vi "PXI-2514 RT Driver VI.vi"(6 "Device Clock":string, 9 "Device Inputs FIFO":refnum<k33>, 10 "Device Outputs FIFO":refnum<k33>, 11 "Device Reference":T1 format="%.0x") -> ()   [LabVIEW 2011, in "PXI-2514 Custom Device.lvlib"]
uses:
  PXI-2514 Custom Device.lvlib
  <vilib>/NI Veristand/Custom Device API/Custom Device Item Ref.ctl
  <vilib>/NI Veristand/Custom Device API/Custom Device Channel Type.ctl
  <vilib>/Platform/TimedLoop/XDataNode/timing_clust.ctl
  <vilib>/Platform/TimedLoop/XDataNode/nitl_modes.ctl
  <vilib>/Platform/TimedLoop/XDataNode/wakeup.ctl
  FIU Global Strings.vi
  <vilib>/NI Veristand/Custom Device API/Get Item Property (String).vi
  <vilib>/Platform/TimedLoop/XDataNode/XDataNode.xnode
  <vilib>/Platform/TimedLoop/XDataNode/XDNodeRunTimeDep.lvlib
  <vilib>/NI Veristand/Custom Device API/Custom Device API.lvlib
panel:
  in  "Status Notifier":refnum<notifier>
  # "Custom Device Template\nv1.0"
  # "Use this template as a starting point for creating a custom device code module. The input controls shown here are specially named controls that the system will use to provide the device loop with data. The controls are not required for the device loop to run. For instance, if the device doesn't produce any output data, then you don't need the Device Outputs FIFO control. If you do use these controls, however, they need to have these exact names to be functional."
  # "The optional status notifier element is used to notify the RT engine of the last state of the custom device, and to indicate the device has completed execution. If this control is not used, a default No Error value is returned to the system when the device finishes execution."
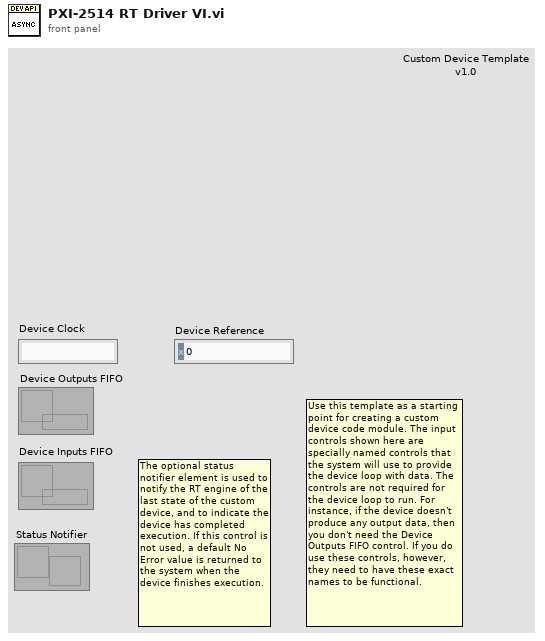
[diagram p1: front panel]
types:
  T1 = typedef "Custom Device API.lvlib/Custom Device Item Ref.ctl" = u64
  T2 = typedef "Custom Device API.lvlib/Custom Device Channel Type.ctl" = enum16{"Input", "Output"}
  T3 = typedef "Custom Device API.lvlib/Custom Device Timed Loop Priority.ctl" = enum32{"Low", "Medium", "High"}
  T4 = typedef "XDNodeRunTimeDep.lvlib/timing_clust.ctl" = cluster{"Expected End [f-1]":u64, "Actual End [f-1]":u64, "Finished Late? [f-1]":bool, "Expected End [i-1]":u64, "Actual End [i-1]":u64, "Finished Late? [i-1]":bool, "Expected Start [i]":u64, "Actual Start [i]":u64, "Expected Start [f]":u64, "Actual Start [f]":u64, "Source Name":string, "Structure Name":string, "Period":i64, "Deadline":i64, "Offset":i64, "Start":i64, "Priority":i32, "Timeout":i32, "Mode":T5, "Wakeup Reason":T6, "Error":errorcluster, "Source Type":string, "Secondary Source Type":string, "Global End Time":u64, "Global Start Time":u64, "Frame Duration":u64, "Iteration Duration":u64, "Assigned CPU":i32, "I/O Scan Engine Mode":u32}
  T5 = typedef "XDNodeRunTimeDep.lvlib/nitl_modes.ctl" = enum32{"No Change", "Process missed periods, maintain original phase", "Discard missed periods, maintain original phase", "Process missed periods, ignore original phase", "Discard missed periods, ignore original phase"}
  T6 = typedef "XDNodeRunTimeDep.lvlib/wakeup.ctl" = enum32{"Normal", "Aborted", "Asynchronous wakeup", "Timing source error", "Timed loop error", "Timeout"}
  T7 = enum16{"Default", "DUT Pass Through", "DUT Open", "DUT Pass Through and FB A", "DUT Pass Through and FB B", "DUT FB A", "DUT FB B"}
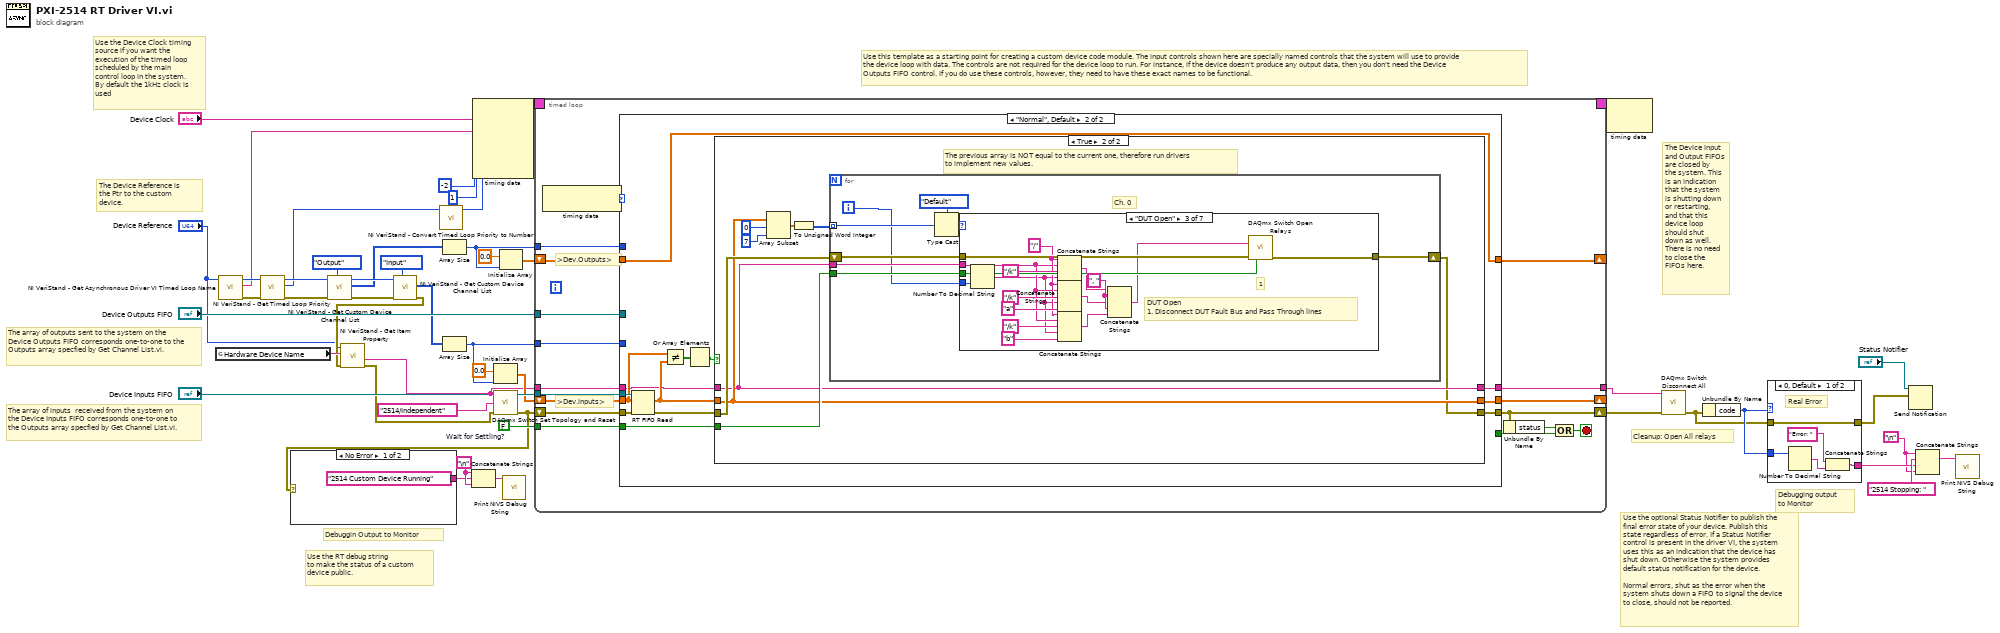
[diagram p0: block diagram]
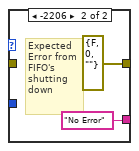
[diagram p2: hidden frame]
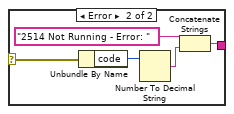
[diagram p3: hidden frame]
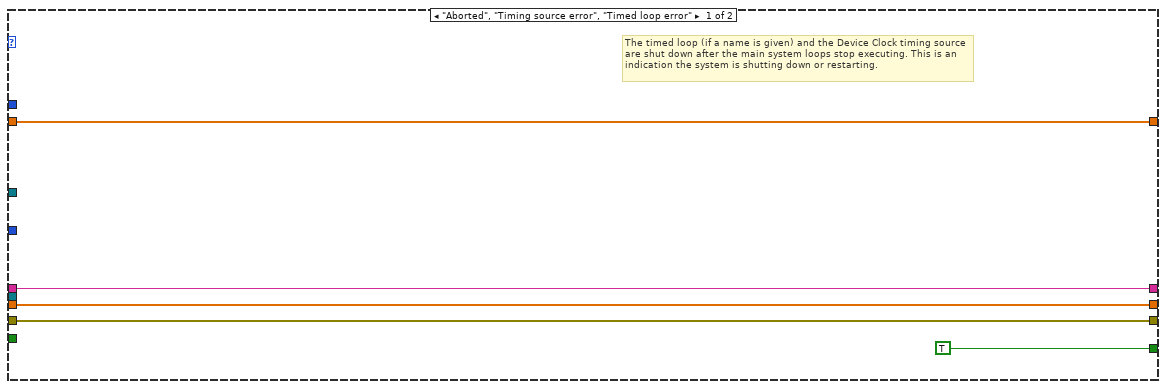
[diagram p4: hidden frame]
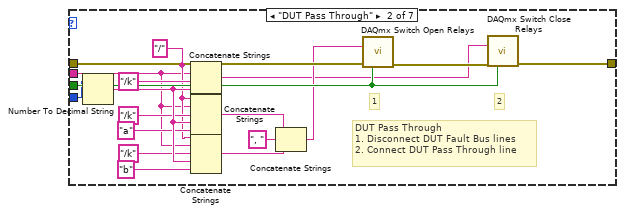
[diagram p7: hidden frame]
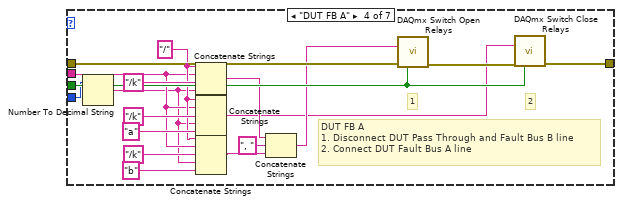
[diagram p8: hidden frame]
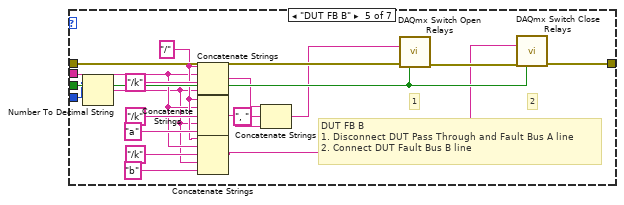
[diagram p9: hidden frame]
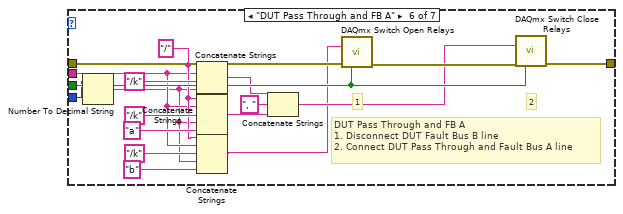
[diagram p10: hidden frame]
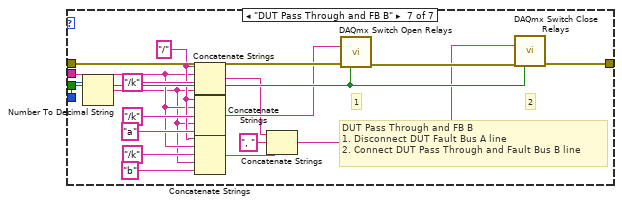
[diagram p11: hidden frame]
diagram:
  w6 = "\n"
  w19 = "\n"
  w22 = FALSE  # Wait for Settling?
  # "Debugging output\nto Monitor"
  # "Debuggin Output to Monitor"
  # "Use the RT debug string\nto make the status of a custom\ndevice public."
  # "Cleanup: Open All relays"
  # "The array of inputs  received from the system on the Device Inputs FIFO corresponds one-to-one to the Outputs array specfied by Get Channel List.vi."
  # "Use the optional Status Notifier to publish the final error state of your device. Publish this state regardless of error. If a Status Notifier control is present in the driver VI, the system uses this as an indication that the device has shut down. Otherwise the system provides default status notification for the device.\n\nNormal errors, shut as the error when the system shuts down a FIFO to signal the device to close, should not be reported."
  # "The Device Input and Output FIFOs are closed by the system. This is an indication that the system is shutting down or restarting, and that this device loop should shut down as well. There is no need to close the FIFOs here."
  # "The array of outputs sent to the system on the Device Outputs FIFO corresponds one-to-one to the Outputs array specfied by Get Channel List.vi."
  # "The Device Reference is\nthe Ptr to the custom device."
  # "Use the Device Clock timing source if you want the execution of the timed loop scheduled by the main control loop in the system. \nBy default the 1kHz clock is used"
  # "Use this template as a starting point for creating a custom device code module. The input controls shown here are specially named controls that the system will use to provide the device loop with data. The controls are not required for the device loop to run. For instance, if the device doesn't produce any output data, then you don't need the Device Outputs FIFO control. If you do use these controls, however, they need to have these exact names to be functional."
  n1 = global read "FIU Global Strings.vi" "Hardware Device Name"() -> (w16:string)
  n2 = call <vilib>:"NI VeriStand - Get Asynchronous Driver VI Timed Loop Name.vi"("Device Ref in"="Device Reference") -> ("error out"=w30:errorcluster, "Device Timed Loop Name"=w36:string, "Device Ref out"=w47:T1)  [unwired: 1 in, 7 out]
  n3 = call <vilib>:"NI VeriStand - Get Timed Loop Priority.vi"("error in (no error)"=w30, "Device Ref in"=w47) -> ("error out"=w31:errorcluster, "Priority"=w27:T3, "Device Ref out"=w32:T1)  [unwired: 7 out]
  n4 = call <vilib>:"NI VeriStand - Get Custom Device Channel List.vi"("Channel Type"=Custom_Device_Channel_Type."Output", "error in (no error)"=w31, "Device Ref in"=w32) -> ("error out"=w35:errorcluster, "Specified Channel Ref List"=w28:T1[], "Device Ref out"=w37:T1)  [unwired: 6 out]
  n5 = call <vilib>:"NI VeriStand - Get Custom Device Channel List.vi"("Channel Type"=Custom_Device_Channel_Type."Input", "error in (no error)"=w35, "Device Ref in"=w37) -> ("error out"=w15:errorcluster, "Specified Channel Ref List"=w29:T1[])  [unwired: 7 out]
  n6 = call-poly <vilib>:"NI VeriStand - Get Item Property.vi"("error in (no error)"=w15, "Property Name"=w16, "Item Ref in"="Device Reference") -> ("error out"=w14:errorcluster, "Value"=w13:string)  [unwired: 5 in, 2 out]
  n7 = call <vilib>:"NI VeriStand - Convert Timed Loop Priority to Number.vi"("Priority"=w27) -> ("Numeric Priority"=w26:i32)  [unwired: 10 out]
  n8 = Array Size(array=w28) -> (size(s)=w33:i32)
  n9 = Array Size(array=w29) -> (size(s)=w23:i32)
  n10 = node-c288("Device Clock", w36, -2 ("Processor"), i64 1 ("Period"), w26) -> (w44:T4)
  n11 = Initialize Array(0.0 ("element"), w23) -> (w39:dbl[])
  n12 = call <vilib>:"DAQmx Switch Set Topology and Reset.vi"("switch device"=w13, "topology name"="2514/Independent" ("string"), "error in"=w14) -> ("error out"=w12:errorcluster)  [unwired: 12 out]
  n13 = case shown="No Error" w12 {
    selector: w12 -> [_ w49]
    tunnel: ["2514 Custom Device Running" ("String to write") w50] -> w18
    frame No Error {
    }
    frame Error {
      n14 = Unbundle By Name(w49) -> ("code"=w53:i32)
      n15 = Number To Decimal String(number=w53) -> (decimal integer string=w51:string)  [unwired: 1 in]
      n16 = Concatenate Strings("2514 Not Running - Error: " ("String to write"), w51) -> (w50:string)
    }
  }
  n17 = Concatenate Strings(w19, w18, w19) -> (w17:string)
  n18 = Initialize Array(0.0 ("element"), w33) -> (w40:dbl[])
  n19 = call "Print NIVS Debug String.vi"("Debug String"=w17) -> ()  [unwired: 9 in, 1 out]
  n20 = timed-loop {
    timing: w44 -> [_]
    timing-out: [_] -> w43
    shift-right: [w68] -> _
    shift-left: w39 -> [w69]
    shift-right: [w61] -> w21
    shift-left: w12 -> [w70]
    shift-right: [w65] -> _
    shift-left: w40 -> [w66]
    tunnel: w33 -> [w62]
    tunnel: "Device Outputs FIFO" -> [w64]
    tunnel: "Device Inputs FIFO" -> [w63]
    tunnel: w23 -> [w57]
    tunnel: w22 -> [w56]
    tunnel: w13 -> [w55]
    tunnel: [w54] -> w20
    stop <- w58 stop-if-true
    # ">Dev.Outputs>"
    # ">Dev.Inputs>"
    n21 = node-c288() -> (w67:T6)  [unwired: 1 out]
    n22 = case shown="\"Normal\", Default" w67 {
      tunnel: w70 -> [w74 w82]
      tunnel: w69 -> [w75 w80]
      tunnel: [w74 w88] -> w61
      tunnel: [w75 w79] -> w68
      tunnel: w66 -> [w73 w78]
      tunnel: [w73 w78] -> w65
      tunnel: w64 -> [_ _]
      tunnel: w63 -> [_ w81]
      tunnel: w62 -> [_ _]
      tunnel: [TRUE _] -> w59
      tunnel: w57 -> [_ _]
      tunnel: w56 -> [_ w87]
      tunnel: w55 -> [w71 w77]
      tunnel: [w71 w76] -> w54
      frame "Aborted", "Timing source error", "Timed loop error" {
        # "The timed loop (if a name is given) and the Device Clock timing source are shut down after the main system loops stop executing. This is an indication the system is shutting down or restarting."
      }
      frame "Normal", Default {
        n23 = RT FIFO Read(0:w81, 1:w80, 3:w82) -> (9:w83:dbl[], 11:w85:errorcluster)  [unwired: 4 out]
        n24 = Not Equal?(x=w80, y=w83) -> (x != y?=w86:bool[])
        n25 = Or Array Elements(Boolean array=w86) -> (logical OR=w84:bool)
        n26 = case shown="True" w84 {
          tunnel: [w90 w92] -> w88
          tunnel: w87 -> [_ w96]
          tunnel: w85 -> [w90 w95]
          tunnel: w83 -> [w91 w94]
          tunnel: [w91 w94] -> w79
          tunnel: w77 -> [w89 w93]
          tunnel: [w89 w93] -> w76
          frame False {
            # "The previous array is equal to the current one, therefore no values have changed and there is no reason\nto run the driver calls again."
          }
          frame True {
            # "The previous array is NOT equal to the current one, therefore run drivers\nto implement new values."
            n27 = Array Subset(array=w94, index=0, length=7) -> (w98:dbl[])
            n28 = To Unsigned Word Integer(number=w98) -> (unsigned 16bit integer=w97:u16[])
            n29 = for {
              tunnel: w97 -> [w108] mode=indexing
              tunnel: w96 -> [w106]
              shift-right: [w105] -> w92
              shift-left: w95 -> [w107]
              tunnel: w93 -> [w104]
              i -> [w103]
              # "Ch. 0"
              n30 = Type Cast(type=T7."Default", x=w108) -> (*(type *) &x=w101:T7)
              n31 = case shown="\"DUT Open\"" w101 {
                tunnel: w107 -> [w109 w126 w144 w161 w179 w197 w215]
                tunnel: [w109 w127 w143 w162 w180 w198 w216] -> w105
                tunnel: w106 -> [_ w124 w142 w159 w177 w195 w213]
                tunnel: w103 -> [_ w115 w129 w156 w174 w192 w210]
                tunnel: w104 -> [_ w110 w133 w149 w167 w185 w203]
                frame Default {
                }
                frame "DUT Pass Through" {
                  w111 = "/" ("string")
                  # "2"
                  # "1"
                  # "DUT Pass Through\n1. Disconnect DUT Fault Bus lines\n2. Connect DUT Pass Through line"
                  n32 = Number To Decimal String(number=w115) -> (decimal integer string=w121:string)  [unwired: 1 out]
                  n33 = Concatenate Strings(w111, w110, "/k", w121) -> (w114:string)
                  n34 = Concatenate Strings(w111, w110, "/k", w121, "a") -> (w113:string)
                  n35 = Concatenate Strings(w111, w110, "/k", w121, "b") -> (w112:string)
                  n36 = Concatenate Strings(w113, ", " ("string"), w112) -> (w122:string)
                  n37 = call <vilib>:"DAQmx Switch Open Relays.vi"("relays"=w122, "error in"=w126, "wait for settling"=w124) -> ("error out"=w125:errorcluster)  [unwired: 12 out]
                  n38 = call <vilib>:"DAQmx Switch Close Relays.vi"("relays"=w114, "error in"=w125, "wait for settling"=w124) -> ("error out"=w127:errorcluster)  [unwired: 12 out]
                }
                frame "DUT Open" {
                  w134 = "/" ("string")
                  w141 = ", " ("string")
                  # "1"
                  # "DUT Open\n1. Disconnect DUT Fault Bus and Pass Through lines"
                  n39 = Number To Decimal String(number=w129) -> (decimal integer string=w128:string)  [unwired: 1 out]
                  n40 = Concatenate Strings(w134, w133, "/k", w128) -> (w132:string)
                  n41 = Concatenate Strings(w134, w133, "/k", w128, "a") -> (w131:string)
                  n42 = Concatenate Strings(w134, w133, "/k", w128, "b") -> (w130:string)
                  n43 = Concatenate Strings(w132, w141, w131, w141, w130) -> (w140:string)
                  n44 = call <vilib>:"DAQmx Switch Open Relays.vi"("relays"=w140, "error in"=w144, "wait for settling"=w142) -> ("error out"=w143:errorcluster)  [unwired: 12 out]
                }
                frame "DUT FB A" {
                  w150 = "/" ("string")
                  # "2"
                  # "1"
                  # "DUT FB A\n1. Disconnect DUT Pass Through and Fault Bus B line\n2. Connect DUT Fault Bus A line"
                  n45 = Number To Decimal String(number=w156) -> (decimal integer string=w148:string)  [unwired: 1 out]
                  n46 = Concatenate Strings(w150, w149, "/k", w148) -> (w147:string)
                  n47 = Concatenate Strings(w150, w149, "/k", w148, "a") -> (w145:string)
                  n48 = Concatenate Strings(w150, w149, "/k", w148, "b") -> (w146:string)
                  n49 = Concatenate Strings(w147, ", " ("string"), w146) -> (w157:string)
                  n50 = call <vilib>:"DAQmx Switch Open Relays.vi"("relays"=w157, "error in"=w161, "wait for settling"=w159) -> ("error out"=w160:errorcluster)  [unwired: 12 out]
                  n51 = call <vilib>:"DAQmx Switch Close Relays.vi"("relays"=w145, "error in"=w160, "wait for settling"=w159) -> ("error out"=w162:errorcluster)  [unwired: 12 out]
                }
                frame "DUT FB B" {
                  w168 = "/" ("string")
                  # "2"
                  # "1"
                  # "DUT FB B\n1. Disconnect DUT Pass Through and Fault Bus A line\n2. Connect DUT Fault Bus B line"
                  n52 = Number To Decimal String(number=w174) -> (decimal integer string=w166:string)  [unwired: 1 out]
                  n53 = Concatenate Strings(w168, w167, "/k", w166) -> (w164:string)
                  n54 = Concatenate Strings(w168, w167, "/k", w166, "a") -> (w163:string)
                  n55 = Concatenate Strings(w168, w167, "/k", w166, "b") -> (w165:string)
                  n56 = Concatenate Strings(w164, ", " ("string"), w163) -> (w175:string)
                  n57 = call <vilib>:"DAQmx Switch Open Relays.vi"("relays"=w175, "error in"=w179, "wait for settling"=w177) -> ("error out"=w178:errorcluster)  [unwired: 12 out]
                  n58 = call <vilib>:"DAQmx Switch Close Relays.vi"("relays"=w165, "error in"=w178, "wait for settling"=w177) -> ("error out"=w180:errorcluster)  [unwired: 12 out]
                }
                frame "DUT Pass Through and FB A" {
                  w186 = "/" ("string")
                  # "2"
                  # "1"
                  # "DUT Pass Through and FB A\n1. Disconnect DUT Fault Bus B line\n2. Connect DUT Pass Through and Fault Bus A line"
                  n59 = Number To Decimal String(number=w192) -> (decimal integer string=w184:string)  [unwired: 1 out]
                  n60 = Concatenate Strings(w186, w185, "/k", w184) -> (w183:string)
                  n61 = Concatenate Strings(w186, w185, "/k", w184, "a") -> (w182:string)
                  n62 = Concatenate Strings(w186, w185, "/k", w184, "b") -> (w181:string)
                  n63 = Concatenate Strings(w183, ", " ("string"), w182) -> (w193:string)
                  n64 = call <vilib>:"DAQmx Switch Open Relays.vi"("relays"=w181, "error in"=w197, "wait for settling"=w195) -> ("error out"=w196:errorcluster)  [unwired: 12 out]
                  n65 = call <vilib>:"DAQmx Switch Close Relays.vi"("relays"=w193, "error in"=w196, "wait for settling"=w195) -> ("error out"=w198:errorcluster)  [unwired: 12 out]
                }
                frame "DUT Pass Through and FB B" {
                  w204 = "/" ("string")
                  # "2"
                  # "1"
                  # "DUT Pass Through and FB B\n1. Disconnect DUT Fault Bus A line\n2. Connect DUT Pass Through and Fault Bus B line"
                  n66 = Number To Decimal String(number=w210) -> (decimal integer string=w202:string)  [unwired: 1 out]
                  n67 = Concatenate Strings(w204, w203, "/k", w202) -> (w200:string)
                  n68 = Concatenate Strings(w204, w203, "/k", w202, "a") -> (w201:string)
                  n69 = Concatenate Strings(w204, w203, "/k", w202, "b") -> (w199:string)
                  n70 = Concatenate Strings(w200, ", " ("string"), w199) -> (w211:string)
                  n71 = call <vilib>:"DAQmx Switch Open Relays.vi"("relays"=w201, "error in"=w215, "wait for settling"=w213) -> ("error out"=w214:errorcluster)  [unwired: 12 out]
                  n72 = call <vilib>:"DAQmx Switch Close Relays.vi"("relays"=w211, "error in"=w214, "wait for settling"=w213) -> ("error out"=w216:errorcluster)  [unwired: 12 out]
                }
              }
            }
          }
        }
      }
    }
    n73 = Unbundle By Name(w61) -> ("status"=w60:bool)
    n74 = Compound Arithmetic op=OR(w60, w59) -> (w58:bool)
  }
  n75 = node-c288(w43) -> ()  [unwired: 1 out]
  n76 = call <vilib>:"DAQmx Switch Disconnect All.vi"("switch device"=w20, "error in"=w21) -> ("error out"=w3:errorcluster)  [unwired: 1 in, 12 out]
  n77 = Unbundle By Name(w3) -> ("code"=w5:i32)
  n78 = case shown="0, Default" w5 {
    tunnel: w3 -> [w224 _]
    tunnel: [w224 errorcluster {"status"=FALSE, "code"=0, "source"=""} ("error out")] -> w10
    tunnel: [w220 "No Error" ("string")] -> w7
    tunnel: w5 -> [w223 _]
    frame 0, Default {
      # "Real Error"
      n79 = Number To Decimal String(number=w223) -> (decimal integer string=w221:string)  [unwired: 1 in]
      n80 = Concatenate Strings("Error: " ("string"), w221) -> (w220:string)
    }
    frame -2206 {
      # "Expected\nError from\nFIFO's \nshutting\ndown"
    }
  }
  n81 = Send Notification(notification=w10, notifier="Status Notifier") -> ()  [unwired: 1 in, 2 out]
  n82 = Concatenate Strings "Concatenate Strings"(w6, "2514 Stopping: " ("string"), w7, w6) -> (w9:string)
  n83 = call "Print NIVS Debug String.vi"("Debug String"=w9) -> ()  [unwired: 9 in, 1 out]
